vi "Path_PPL Folder.vi"() -> (2 "Path Length":i32, 3 "Data Folder Path":path)   [LabVIEW 2020, in "ClassLoader.lvlib"]
doc: "Returns path to the PPL folder. PPLs are assumed to be in a single folder next to each other.\nIf not called from a PPL the VI returns the data-folder."
uses:
  ClassLoader.lvlib
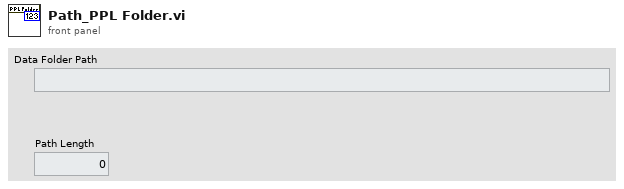
[diagram p1: front panel]
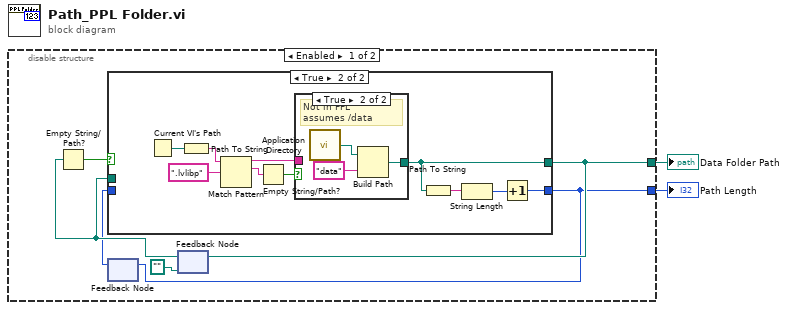
[diagram p0: block diagram]
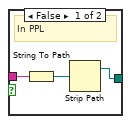
[diagram p3: hidden frame]
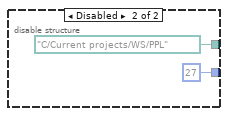
[diagram p4: hidden frame]
diagram:
  n1 = disable-structure shown="Enabled" {
    disable-tunnel: [w6 path "C:/Current projects/WS/PPL" ("path")] -> w2
    disable-tunnel: [w3 27] -> w1
    frame Enabled {
      n2 = feedback #1() -> (w4:i32)  [unwired: 1 in]
      n3 = feedback #2(path "") -> (w5:path)
      n4 = Empty String/Path?(string/path=w5) -> (empty?=w7:bool)
      n5 = case shown="True" w7 {
        tunnel: [w10 w12] -> w6
        tunnel: w5 -> [w10 _]
        tunnel: [w9 w11] -> w3
        tunnel: w4 -> [w9 _]
        frame False {
        }
        frame True {
          n6 = Current VI's Path() -> (path=w20:path)
          n7 = Path To String(path=w20) -> (string=w19:string)
          n8 = Match Pattern(string=w19, regular expression=".lvlibp") -> (before substring=w17:string, match substring=w16:string)  [unwired: 1 in, 2 out]
          n9 = Empty String/Path?(string/path=w16) -> (empty?=w15:bool)
          n10 = case shown="True" w15 {
            tunnel: [w23 w24] -> w12
            tunnel: w17 -> [w22 _]
            frame False {
              # "In PPL"
              n11 = String To Path(string=w22) -> (path=w21:path)
              n12 = Strip Path(path=w21) -> (stripped path=w23:path)  [unwired: 1 out]
            }
            frame True {
              # "Not in PPL assumes /data"
              n13 = call <vilib>:"Application Directory.vi"() -> ("Application Directory"=w26:path)
              n14 = Build Path(base path=w26, name or relative path="data") -> (appended path=w24:path)
            }
          }
          n15 = Path To String(path=w12) -> (string=w14:string)
          n16 = String Length(string=w14) -> (length=w13:i32)
          n17 = Increment(x=w13) -> (x+1=w11:i32)
        }
      }
      n18 = feedback-in #1(w3) -> ()
      n19 = feedback-in #2(w6) -> ()
    }
    frame Disabled {
    }
  }
  "Data Folder Path" <- w2
  "Path Length" <- w1
